vi "Serial Device setup.vi"(8 "error in (no error)":errorcluster) -> (0 "error out":errorcluster, 3 "Module ID":i32)   [LabVIEW 2020]
doc: "_____\nCreated using Delacor QMH Event Scripter 5.0.0.112."
uses:
  Libraries/Serial Device/Serial Device.lvlib
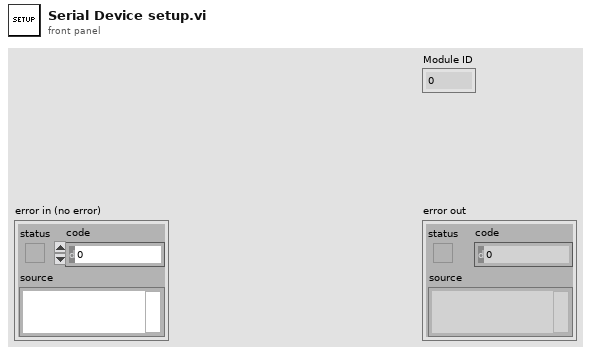
[diagram p1: front panel]
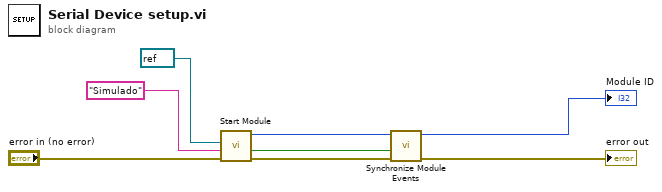
[diagram p0: block diagram]
diagram:
  n1 = call "Start Module.vi"("error in (no error)"="error in (no error)", "Device"="Simulado", "VISA Com Port"=refnum<visa-resource-name> refnum) -> ("error out"=w7:errorcluster, "Wait for Event Sync?"=w3:bool, "Module ID"=w4:i32)  [unwired: 5 in, 1 out]
  n2 = call "Synchronize Module Events.vi"("error in (no error)"=w7, "Wait for Event Sync?"=w3, "Module ID"=w4) -> ("error out"=→"error out":errorcluster, "Module ID (dup)"=→"Module ID":i32)  [unwired: 7 in]
